vi "DAQNavi Read (Digital 1D U8 NChan 1Samp).vi"(8 "error in (no error)":errorcluster, 10 "timeout":dbl=10.0 format="%0.2f", 11 "task in":i32) -> (0 "error out":errorcluster, 2 "data":u8[](array[numeric]), 3 "task out":i32)   [LabVIEW 2020]
uses:
  DAQNavi_LV.dll
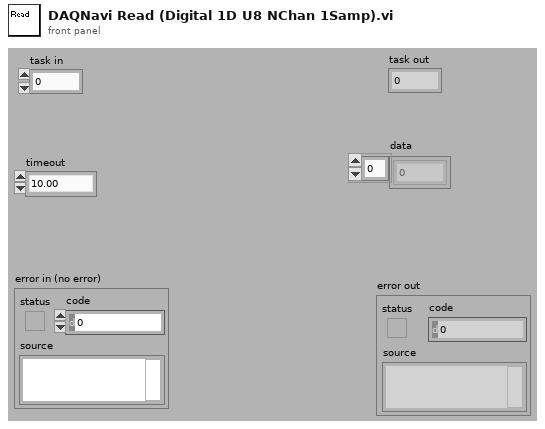
[diagram p1: front panel]
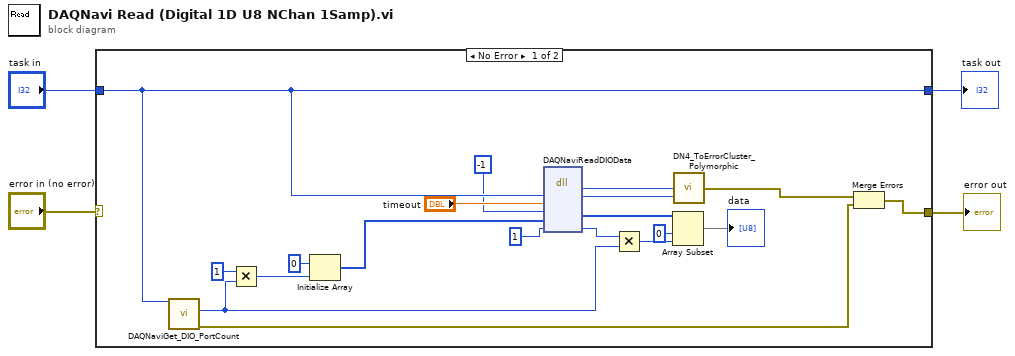
[diagram p0: block diagram]
diagram:
  n1 = case shown="No Error" "error in (no error)" {
    selector: "error in (no error)" -> [_ w24]
    tunnel: "task in" -> [w17 w25]
    tunnel: [w17 w25] -> w2
    tunnel: [w14 w24] -> w1
    frame No Error {
      n2 = call "DAQNaviGet_DIO_PortCount.vi"("task in"=w17) -> ("error out"=w15:errorcluster, "port count"=w11:i32)  [unwired: 1 in, 8 out]
      n3 = Multiply(x=1 ("y"), y=w11) -> (x*y=w18:i32)
      n4 = Initialize Array(u8 0 ("element"), w18) -> (w9:u8[])
      n5 = dll-call lib="DAQNavi_LV.dll" fn="DAQNaviReadDIOData"("taskID"=w17, "timeout"="timeout", "portBit"=-1, "portData"=w9, "samples"=1) -> ("return type"=w20:i32, "taskID"=w6:i32, "portData"=w8:u8[], "samples"=w12:i32)  [unwired: 5 in, 2 out]
      n6 = Multiply(x=w12, y=w11) -> (x*y=w10:i32)
      n7 = Array Subset(array=w8, index=0, length=w10) -> (→"data":u8[])
      n8 = call "DN4_ToErrorCluster_Polymorphic.vi"("task id"=w6, "error code"=w20) -> ("error out"=w16:errorcluster)  [unwired: 3 out]
      n9 = Merge Errors(w16, w15) -> (w14:errorcluster)
    }
    frame Error {
    }
  }
  "task out" <- w2
  "error out" <- w1
